vi "Build IP address string.vi"(4 "IP address":string) -> (1 "IP Name":string)   [LabVIEW 2020]
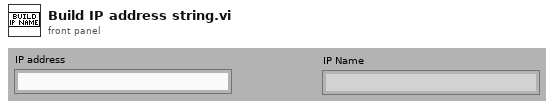
[diagram p1: front panel]
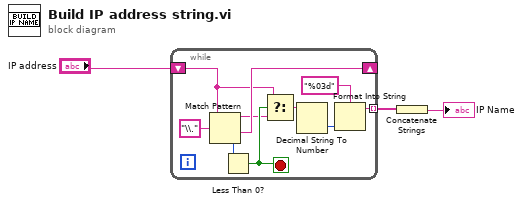
[diagram p0: block diagram]
diagram:
  n1 = while {
    shift-right: [w7] -> _
    shift-left: "IP address" -> [w4]
    tunnel: [w12] -> w2 mode=indexing
    stop <- w8 stop-if-true
    n2 = Match Pattern(string=w4, regular expression="\\.") -> (before substring=w6:string, after substring=w7:string, offset past match=w9:i32)  [unwired: 1 in, 1 out]
    n3 = Less Than 0?(x=w9) -> (x < 0?=w8:bool)
    n4 = Select(t=w4, s=w8, f=w6) -> (s? t:f=w5:string)
    n5 = Decimal String To Number(string=w5) -> (number=w11:i32)  [unwired: 2 in, 1 out]
    n6 = Format Into String(format string="%03d", w11) -> (resulting string=w12:string)  [unwired: 2 in, 1 out]
  }
  n7 = Concatenate Strings(w2) -> (→"IP Name":string)
